vi "BB_Aspect_ratio_score.vi"(8 "Equivalent Rect Short":dbl, 9 "Equivalent Rect Long":dbl, 10 "Height":dbl, 11 "Width":dbl) -> (1 "Verticle":dbl, 2 "Middle":dbl, 3 "High":dbl)   [LabVIEW 2015]
doc: "Compare the ratio of the rectangle to that of the expected target. Score is in percent.\n\nSince inputs are particle measurements, the diagram doesn't expect to receive zero or negative values for either input."
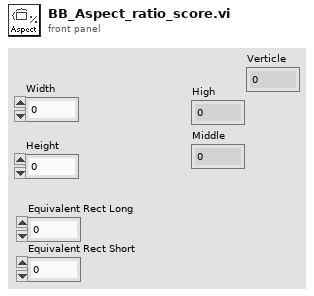
[diagram p1: front panel]
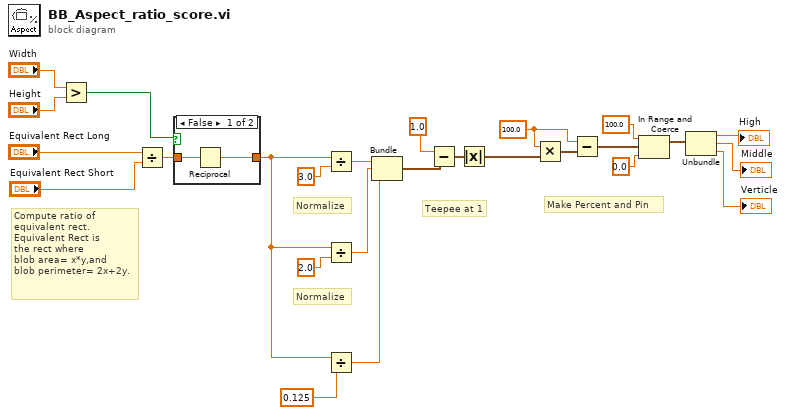
[diagram p0: block diagram]
diagram:
  w20 = 100.0 ("x/y")
  # "Make Percent and Pin"
  # "Teepee at 1"
  # "Normalize"
  # "Normalize"
  # "Compute ratio of\nequivalent rect.\nEquivalent Rect is\nthe rect where\nblob area= x*y,and\nblob perimeter= 2x+2y."
  n1 = Greater?(x="Width", y="Height") -> (0:w5:bool)
  n2 = Divide(x="Equivalent Rect Long", y="Equivalent Rect Short") -> (x/y=w6:dbl)
  n3 = case shown="False" w5 {
    tunnel: w6 -> [w28 w29]
    tunnel: [w27 w29] -> w3
    frame False {
      n4 = Reciprocal(x=w28) -> (1/x=w27:dbl)
    }
    frame True {
    }
  }
  n5 = Divide(x=w3, y=3.0) -> (x/y=w14:dbl)
  n6 = Divide(x=w3, y=2.0) -> (x/y=w13:dbl)
  n7 = Divide(x=w3, y=0.125) -> (x/y=w2:dbl)
  n8 = Bundle(w14, w13, w2) -> (w12:cluster{dbl, dbl, dbl})  [unwired: 1 in]
  n9 = Subtract(x=1.0 ("y"), y=w12) -> (x-y=w18:cluster{dbl, dbl, dbl})
  n10 = Absolute Value(x=w18) -> (abs(x)=w21:cluster{dbl, dbl, dbl})
  n11 = Multiply(x=w20, y=w21) -> (x*y=w22:cluster{dbl, dbl, dbl})
  n12 = Subtract(x=w20, y=w22) -> (x-y=w17:cluster{dbl, dbl, dbl})
  n13 = In Range and Coerce(upper limit=100.0, x=w17, lower limit=0.0) -> (coerced(x)=w11:cluster{dbl, dbl, dbl})  [unwired: 1 out]
  n14 = Unbundle(w11) -> (→"High":dbl, →"Middle":dbl, →"Verticle":dbl)
